vi "Calculate nAT per B.vi"(11 "Scan Parameters":T1={"# Scan"={"#Ascan"=400, "#Bscan"=400}, "# Rpt"={"#ARpt"=1, "#BRpt"=1}, "Aline Rate"=2, "# Extra"={"# ARpt_extra"=5, "#Brtn_extra"=60}} {"Aline Rate" items=["76 KHz", "146 KHz", "76 KHz", "28 KHz", "10 KHz"]}) -> (1 "nA per B":i32, 2 "Brtn_extra/2":i32, 3 "nAT per B":i32)   [LabVIEW 2017]
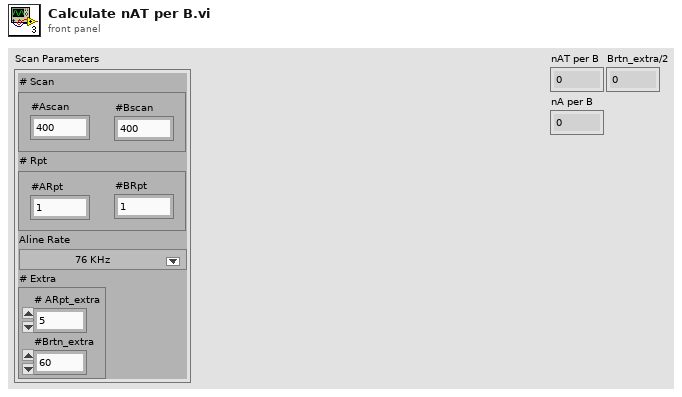
[diagram p1: front panel]
types:
  T1 = cluster{"# Scan":cluster{"#Ascan":i32, "#Bscan":i32}, "# Rpt":cluster{"#ARpt":i32, "#BRpt":i32}, "Aline Rate":u16, "# Extra":cluster{"# ARpt_extra":i32, "#Brtn_extra":i32}}
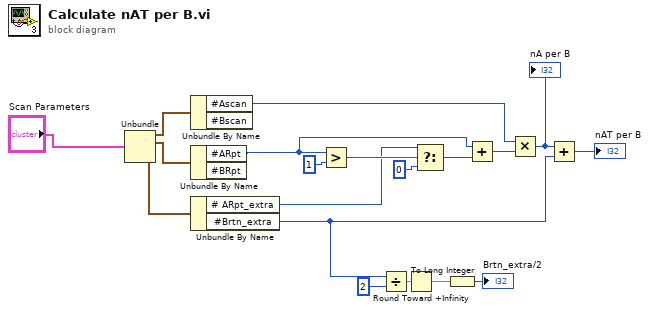
[diagram p0: block diagram]
diagram:
  n1 = Unbundle("Scan Parameters") -> ("# Scan"=w10:cluster{"#Ascan":i32, "#Bscan":i32}, "# Rpt"=w18:cluster{"#ARpt":i32, "#BRpt":i32}, "# Extra"=w13:cluster{"# ARpt_extra":i32, "#Brtn_extra":i32})  [unwired: 1 out]
  n2 = Unbundle By Name(w10) -> ("#Ascan"=w8:i32)  [unwired: 1 out]
  n3 = Unbundle By Name(w18) -> ("#ARpt"=w11:i32)  [unwired: 1 out]
  n4 = Unbundle By Name(w13) -> ("# ARpt_extra"=w12:i32, "#Brtn_extra"=w5:i32)
  n5 = Greater?(x=w11, y=1) -> (0:w16:bool)
  n6 = Divide(x=w5, y=2) -> (x/y=w3:dbl)
  n7 = Round Toward +Infinity(x=w3) -> (ceil(x): smallest int >= x=w2:dbl)
  n8 = Select(t=w12, s=w16, f=0) -> (s? t:f=w14:i32)
  n9 = To Long Integer(number=w2) -> (32bit integer=→"Brtn_extra/2":i32)
  n10 = Add(x=w11, y=w14) -> (x+y=w9:i32)
  n11 = Multiply(x=w8, y=w9) -> (x*y=w7:i32)
  "nA per B" <- w7
  n12 = Add(x=w7, y=w5) -> (x+y=→"nAT per B":i32)
